vi "classify error.vi"(8 "error to classify":errorcluster, 10 "attempt recovery?":bool, 11 "fixed channel runtime in":refnum<class "control module runtime.lvclass">) -> (0 "classified error":errorcluster, 2 "error classification":T1, 3 "fixed channel runtime out":refnum<class "control module runtime.lvclass">)   [LabVIEW 2013, in "control module runtime.lvclass"]
doc: "Allows a module to classify an error generated at any point during execution. This <b>error classification</b> can then be used by calling code to determine if execution can continue. In addition, this function can be used to allow a component to clear an error, convert an error to a warning, or attempt to recover from an error. Recovery may be attempted only if <b>attempt recovery?</b> is true."
uses:
  control module runtime.lvclass
  <vilib>/NI/Tag Bus Module Framework/runtime/error classification.ctl
  <vilib>/NI/Tag Bus Module Framework/runtime/TBM module execution interface.lvclass
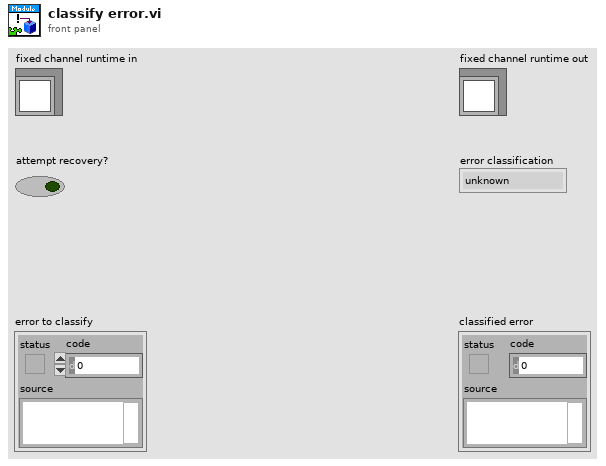
[diagram p1: front panel]
types:
  T1 = typedef "TBM module execution interface.lvclass/error classification.ctl" = enum16{"unknown", "none", "trivial", "recoverable", "critical"}
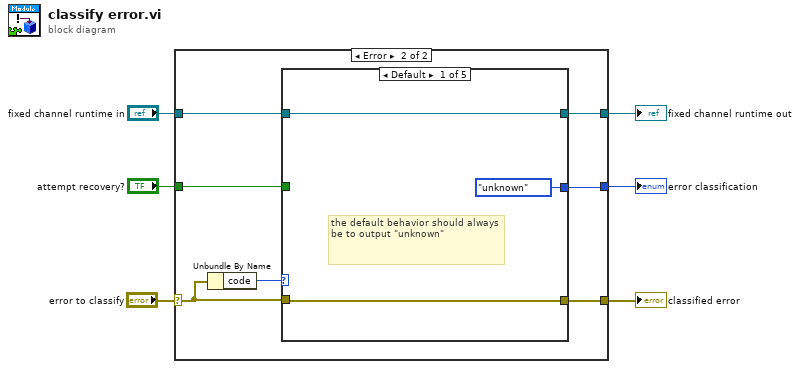
[diagram p0: block diagram]
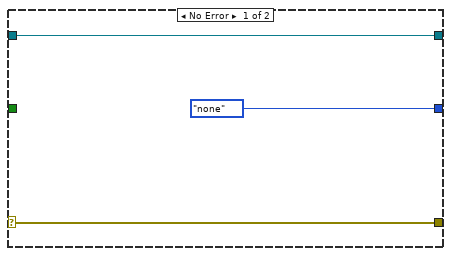
[diagram p2: hidden frame]
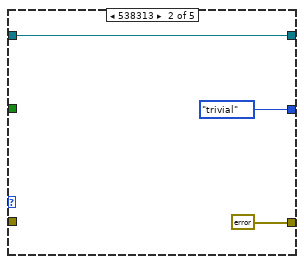
[diagram p3: hidden frame]
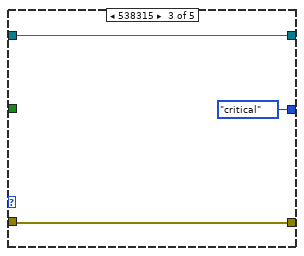
[diagram p4: hidden frame]
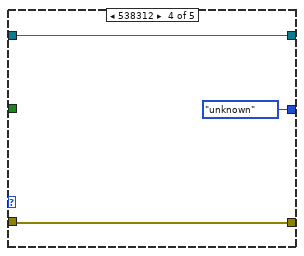
[diagram p5: hidden frame]
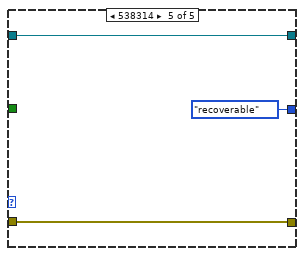
[diagram p6: hidden frame]
diagram:
  n1 = case shown="Error" "error to classify" {
    selector: "error to classify" -> [w8 w15]
    tunnel: "attempt recovery?" -> [_ w10]
    tunnel: [w9 w11] -> w4
    tunnel: "fixed channel runtime in" -> [w9 w12]
    tunnel: [w8 w14] -> w2
    tunnel: [error_classification."none" ("error classification") w13] -> w1
    frame No Error {
    }
    frame Error {
      n2 = Unbundle By Name(w15) -> ("code"=w16:i32)
      n3 = case shown="Default" w16 {
        tunnel: w15 -> [w17 _ w23 w26 w31]
        tunnel: [w17 errorcluster {"status"=FALSE, "code"=0, "source"=""} ("error constant") w23 w26 w31] -> w14
        tunnel: [error_classification."unknown" ("error classification") error_classification."trivial" ("error classification") error_classification."critical" ("error classification") error_classification."unknown" ("error classification") error_classification."recoverable" ("error classification")] -> w13
        tunnel: w12 -> [w18 w20 w25 w28 w29]
        tunnel: [w18 w20 w25 w28 w29] -> w11
        tunnel: w10 -> [_ _ _ _ _]
        frame Default {
          # "the default behavior should always be to output \"unknown\""
        }
        frame 538313 {
        }
        frame 538315 {
        }
        frame 538312 {
        }
        frame 538314 {
        }
      }
    }
  }
  "fixed channel runtime out" <- w4
  "error classification" <- w1
  "classified error" <- w2
